vi "subParseXMLString.vi"(9 "Parents in":string[](array[string]), 11 "input string":string) -> (1 "Parents":string[](array[string]), 2 "Value":string, 3 "Parameter":string, 5 "Parent?":bool)   [LabVIEW 2020, in "CommonHelpers.lvlib"]
uses:
  CommonHelpers.lvlib
  <vilib>/regexp/Match Regular Expression.xnode
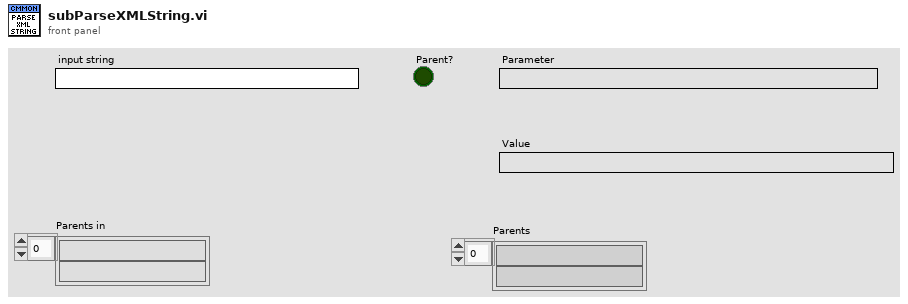
[diagram p1: front panel]
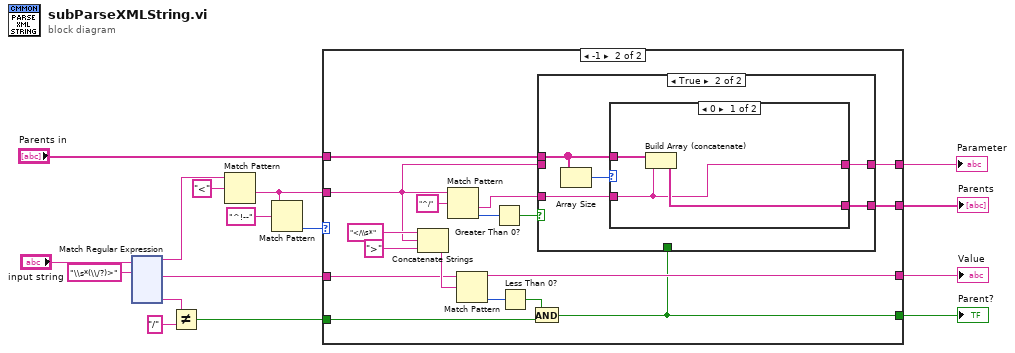
[diagram p0: block diagram]
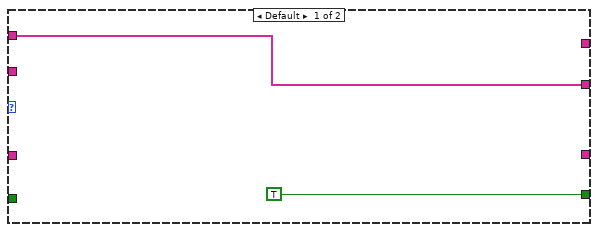
[diagram p2: hidden frame]
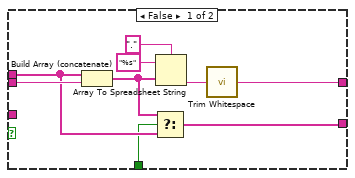
[diagram p3: hidden frame]
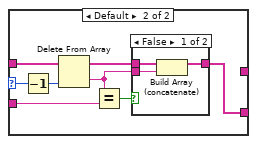
[diagram p4: hidden frame]
diagram:
  n1 = xnode "Match Regular Expression"("input string"="input string", "regular expression"="\\s*(\\/?)>") -> ("before match"=w14:string, "after match"=w13:string, "submatch 1"=w12:string)  [unwired: 4 in, 3 out]
  n2 = Not Equal?(x=w12, y="/") -> (x != y?=w6:bool)
  n3 = Match Pattern(string=w14, regular expression="<") -> (after substring=w2:string)  [unwired: 1 in, 3 out]
  n4 = Match Pattern(string=w2, regular expression="^!--") -> (offset past match=w1:i32)  [unwired: 1 in, 3 out]
  n5 = case shown="-1" w1 {
    tunnel: w13 -> [_ w33]
    tunnel: "Parents in" -> [w18 w32]
    tunnel: [_ w31] -> w9
    tunnel: [_ w25] -> w7
    tunnel: w6 -> [_ w24]
    tunnel: [w18 w23] -> w5
    tunnel: [TRUE w22] -> w4
    tunnel: w2 -> [_ w19]
    frame Default {
    }
    frame -1 {
      n6 = Concatenate Strings("</\\s*" ("t"), w19, ">" ("string")) -> (w34:string)
      n7 = Match Pattern(string=w19, regular expression="^/") -> (after substring=w26:string, offset past match=w28:i32)  [unwired: 1 in, 2 out]
      n8 = Match Pattern(string=w33, regular expression=w34) -> (before substring=w25:string, offset past match=w21:i32)  [unwired: 1 in, 2 out]
      n9 = Greater Than 0?(x=w28) -> (x > 0?=w27:bool)
      n10 = Less Than 0?(x=w21) -> (x < 0?=w20:bool)
      n11 = And(x=w20, y=w24) -> (x .and. y?=w22:bool)
      n12 = case shown="True" w27 {
        tunnel: w32 -> [w40 w49]
        tunnel: [w36 w45] -> w31
        tunnel: w19 -> [w43 _]
        tunnel: w26 -> [_ w48]
        tunnel: [w38 w47] -> w23
        tunnel: w22 -> [w37 _]
        frame False {
          n13 = Build Array (concatenate)(w40, w43) -> (w39:string[])
          n14 = Select(t=w39, s=w37, f=w40) -> (s? t:f=w38:string[])
          n15 = Array To Spreadsheet String(delimiter (Tab)=".", array=w39, 3:"%s" ("format string")) -> (spreadsheet string=w44:string)
          n16 = call <vilib>:"Trim Whitespace.vi"("string"=w44) -> ("trimmed string"=w36:string)  [unwired: 1 in]
        }
        frame True {
          n17 = Array Size(array=w49) -> (size(s)=w46:i32)
          n18 = case shown="0" w46 {
            selector: w46 -> [_ w53]
            tunnel: w49 -> [w52 w60]
            tunnel: w48 -> [w50 w56]
            tunnel: [w51 w54] -> w47
            tunnel: [w50 _] -> w45
            frame 0 {
              n19 = Build Array (concatenate)(w52, w50) -> (w51:string[])
            }
            frame Default {
              n20 = Decrement(x=w53) -> (x-1=w55:i32)
              n21 = Delete From Array(array=w60, index=w55) -> (deleted portion=w57:string, array with subset deleted=w59:string[])  [unwired: 1 in]
              n22 = Equal?(x=w57, y=w56) -> (x = y?=w58:bool)
              n23 = case shown="False" w58 {
                tunnel: w59 -> [w63 w64]
                tunnel: [w61 w64] -> w54
                tunnel: w57 -> [w62 _]
                frame False {
                  n24 = Build Array (concatenate)(w63, w62) -> (w61:string[])
                }
                frame True {
                }
              }
            }
          }
        }
      }
    }
  }
  "Parameter" <- w9
  "Value" <- w7
  "Parent?" <- w4
  "Parents" <- w5
